vi "Merge Call Library Errors.vi"(4 "Call Library Error":errorcluster, 6 "Return Value":i32, 8 "error in":errorcluster) -> (0 "error out":errorcluster)   [LabVIEW 2020, in "G-Embedded-Python-Interpreter-Toolkit.lvlib"]
uses:
  G-Embedded-Python-Interpreter-Toolkit.lvlib
  <vilib>/Utility/error.llb/Error Cluster From Error Code.vi
  <vilib>/ErrorRing/Error Ring.xnode
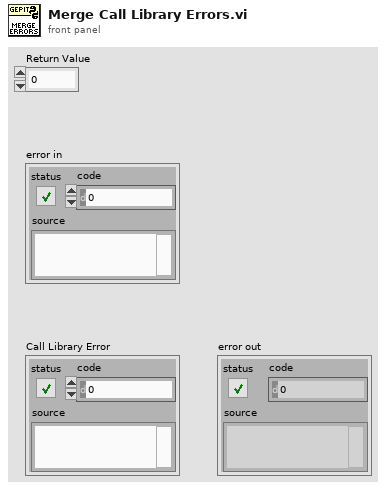
[diagram p1: front panel]
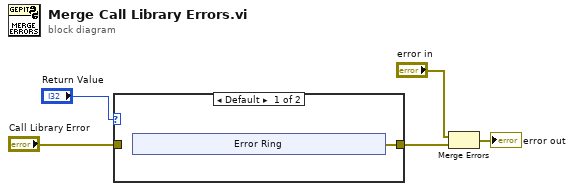
[diagram p0: block diagram]
diagram:
  n1 = case shown="Default" "Return Value" {
    tunnel: "Call Library Error" -> [_ w12]
    tunnel: [w6 w12] -> w3
    frame Default {
      n2 = xnode "Error Ring"() -> ("error out"=w6:errorcluster)
    }
    frame 0 {
    }
  }
  n3 = Merge Errors("error in", w3) -> (→"error out":errorcluster)
